vi "PAN_SeparateCmds.vi"(10 "cmd in":string) -> (2 "cmds out":string[](array[string]))   [LabVIEW 2016]
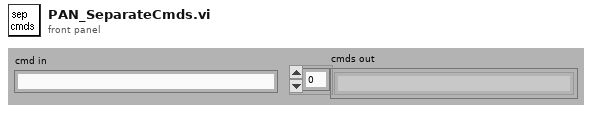
[diagram p1: front panel]
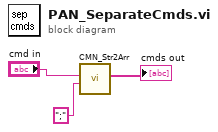
[diagram p0: block diagram]
diagram:
  n1 = call "CMN_Str2Arr.vi"("separator"=";", "string in"="cmd in") -> ("Array out"=→"cmds out":string[])  [unwired: 2 in, 7 out]
